vi "I2C.Config.vi"(8 "error in":errorcluster, 9 "msDelay (Optional)":u8, 11 "comport in":refnum<visa-resource-name>) -> (0 "error out":errorcluster, 3 "comport out":refnum<visa-resource-name>)   [LabVIEW 2020, in "FirmataClient.lvlib"]
doc: "Configures UUT's I2C port running on its board"
uses:
  FirmataClient.lvlib
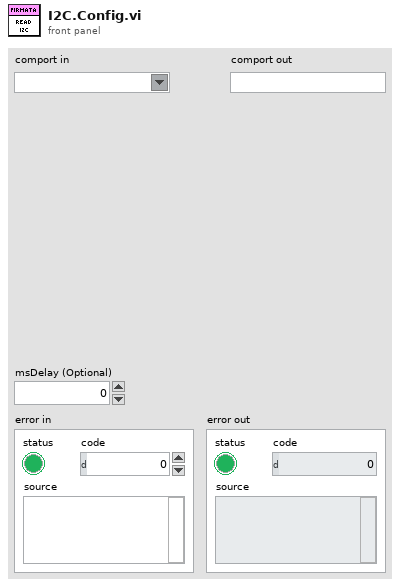
[diagram p1: front panel]
types:
  T1 = typedef "FirmataClient.lvlib/FirmataProtocolConstants.ctl" = u16
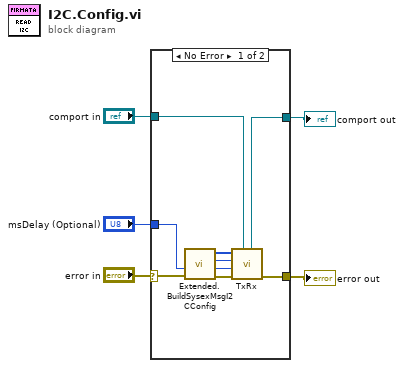
[diagram p0: block diagram]
diagram:
  n1 = case shown="No Error" "error in" {
    selector: "error in" -> [w8 w16]
    tunnel: [w7 w16] -> w4
    tunnel: [w10 w15] -> w2
    tunnel: "comport in" -> [w9 w15]
    tunnel: "msDelay (Optional)" -> [w6 _]
    frame No Error {
      n2 = call "Extended.BuildSysexMsgI2CConfig.vi"("error in"=w8, "msDelay (Optional)"=w6) -> ("error out"=w14:errorcluster, "ReplyLength"=w11:i32, "ReplyFirstByte"=w12:T1, "GetPinStateMessage"=w13:u8[])  [unwired: 6 in]
      n3 = call "TxRx.vi"("comport in"=w9, "error in"=w14, "Expected Reply Length"=w11, "ReplyFirstByte"=w12, "MessageToSend"=w13) -> ("error out"=w7:errorcluster, "comport out"=w10:refnum<visa-resource-name>)  [unwired: 2 in, 3 out]
    }
    frame Error {
    }
  }
  "error out" <- w4
  "comport out" <- w2
